vi "DAQNavi Create Channel(AI-Current).vi"(0 "task in":i32=-1, 5 "physical channels":string="DemoDevice,BID#0/ai0", 7 "signal type":string(combo)="Omit", 9 "value range":string(combo)="Omit", 11 "error in (no error)":errorcluster) -> (4 "task out":i32, 15 "error out":errorcluster)   [LabVIEW 2020]
uses:
  DAQNavi_LV.dll
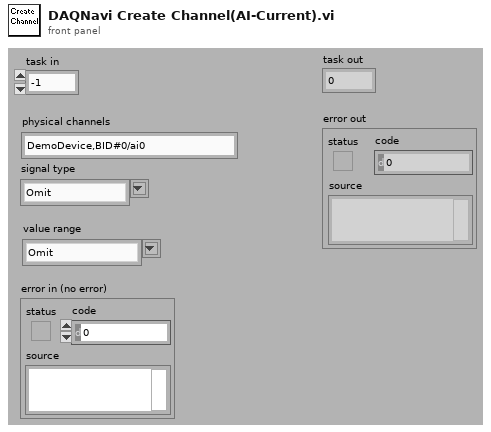
[diagram p1: front panel]
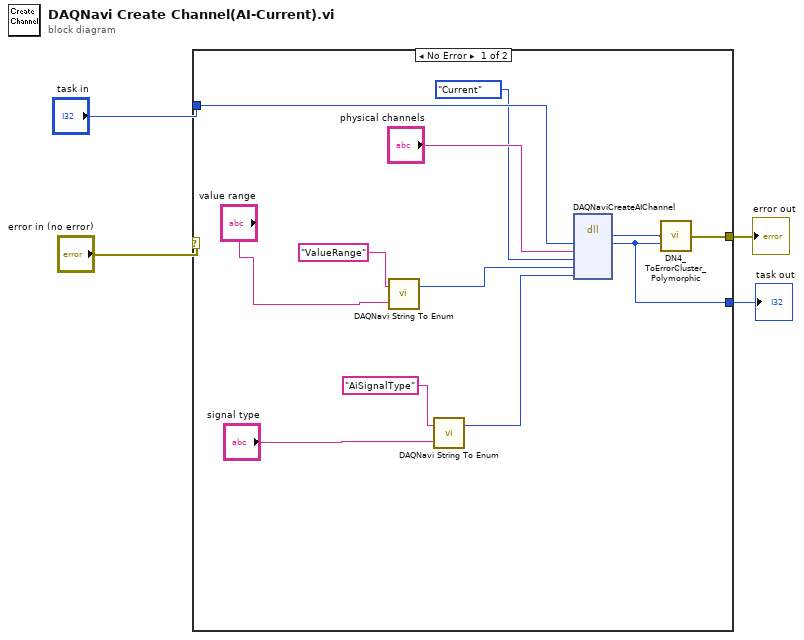
[diagram p0: block diagram]
diagram:
  n1 = case shown="No Error" "error in (no error)" {
    selector: "error in (no error)" -> [_ w17]
    tunnel: "task in" -> [w16 w18]
    tunnel: [w10 w17] -> w2
    tunnel: [w9 w18] -> w1
    frame No Error {
      n2 = call "DAQNavi String To Enum.vi"("enumString"="value range", "enumTypeName"="ValueRange") -> ("enumValue"=w12:i32)  [unwired: 1 out]
      n3 = call "DAQNavi String To Enum.vi"("enumString"="signal type", "enumTypeName"="AiSignalType") -> ("enumValue"=w13:i32)  [unwired: 1 out]
      n4 = dll-call lib="DAQNavi_LV.dll" fn="DAQNaviCreateAIChannel"("taskID"=w16, "physicalChannel"="physical channels", "type"=enum32{"Voltage", "Temperature", "Current"}."Current", "valueRange"=w12, "signalType"=w13) -> ("return type"=w11:i32, "taskID"=w9:i32)  [unwired: 6 in, 3 out]
      n5 = call "DN4_ToErrorCluster_Polymorphic.vi"("task id"=w9, "error code"=w11) -> ("error out"=w10:errorcluster)  [unwired: 3 out]
    }
    frame Error {
    }
  }
  "error out" <- w2
  "task out" <- w1
